vi "8-i-dist.vi"(1 "n":u32, 2 "i":i32) -> (0 "R(i) médian obs_n":dbl)   [LabVIEW 2010, in "lv_02.lvlib"]
uses:
  lv_02.lvlib
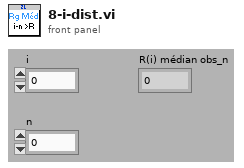
[diagram p1: front panel]
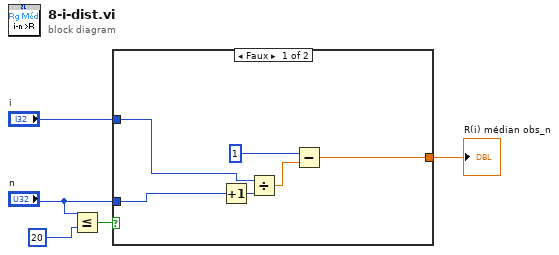
[diagram p0: block diagram]
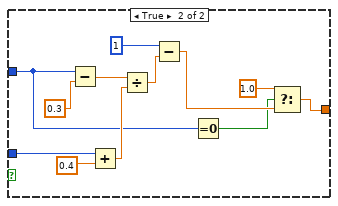
[diagram p2: hidden frame]
diagram:
  n1 = Less Or Equal?(x="n", y=u32 20) -> (x <= y?=w3:bool)
  n2 = case shown="Faux" w3 {
    tunnel: "n" -> [w10 w23]
    tunnel: [w9 w19] -> w5
    tunnel: "i" -> [w11 w12]
    frame False {
      n3 = Increment(x=w10) -> (x+1=w7:u32)
      n4 = Divide(x=w11, y=w7) -> (x/y=w6:dbl)
      n5 = Subtract(x=1, y=w6) -> (x-y=w9:dbl)
    }
    frame True {
      n6 = Subtract(x=w12, y=0.3) -> (x-y=w16:dbl)
      n7 = Add(x=w23, y=0.4) -> (x+y=w14:dbl)
      n8 = Divide(x=w16, y=w14) -> (x/y=w21:dbl)
      n9 = Subtract(x=1, y=w21) -> (x-y=w22:dbl)
      n10 = Equal To 0?(x=w12) -> (x = 0?=w17:bool)
      n11 = Select(t=1.0 ("cas vrai"), s=w17, f=w22) -> (s? t:f=w19:dbl)
    }
  }
  "R(i) médian obs_n" <- w5
